vi "Switch Tables.vi"(6 "New Table Name":string, 8 "error in (no error)":errorcluster, 9 "Column Name":string, 10 "Old Table Name":string, 11 "Data.PG":refnum<class "LV-Data.PGSQL.lvclass">) -> (0 "error out":errorcluster, 3 "Data.PG out":refnum<class "LV-Data.PGSQL.lvclass">)   [LabVIEW 2019, in "LV-Data.PGSQL.lvclass"]
uses:
  LV-Data.PGSQL.lvclass
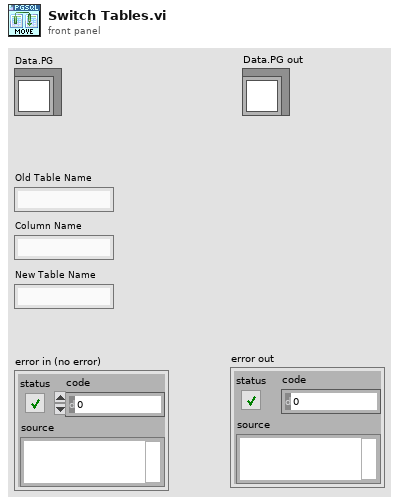
[diagram p1: front panel]
types:
  T1 = enum16{"max points", "1 second", "5 seconds", "10 seconds", "30 seconds", "1 minute", "5 minutes", "10 minutes", "30 minutes", "1 hour", "5 hours", "10 hours", "30 hours"}
  T2 = cluster{"start timestamp":timestamp, "stop timestamp":timestamp}
  T3 = typedef "LV-Data.PGSQL.lvclass/Time.Datatype--enum.ctl" = enum16{"timestamp without time zone", "timestamp with time zone"}
  T4 = typedef "LV-Data.PGSQL.lvclass/Datatypes--enum.ctl" = enum16{"double", "string", "json", "integer", "boolean"}
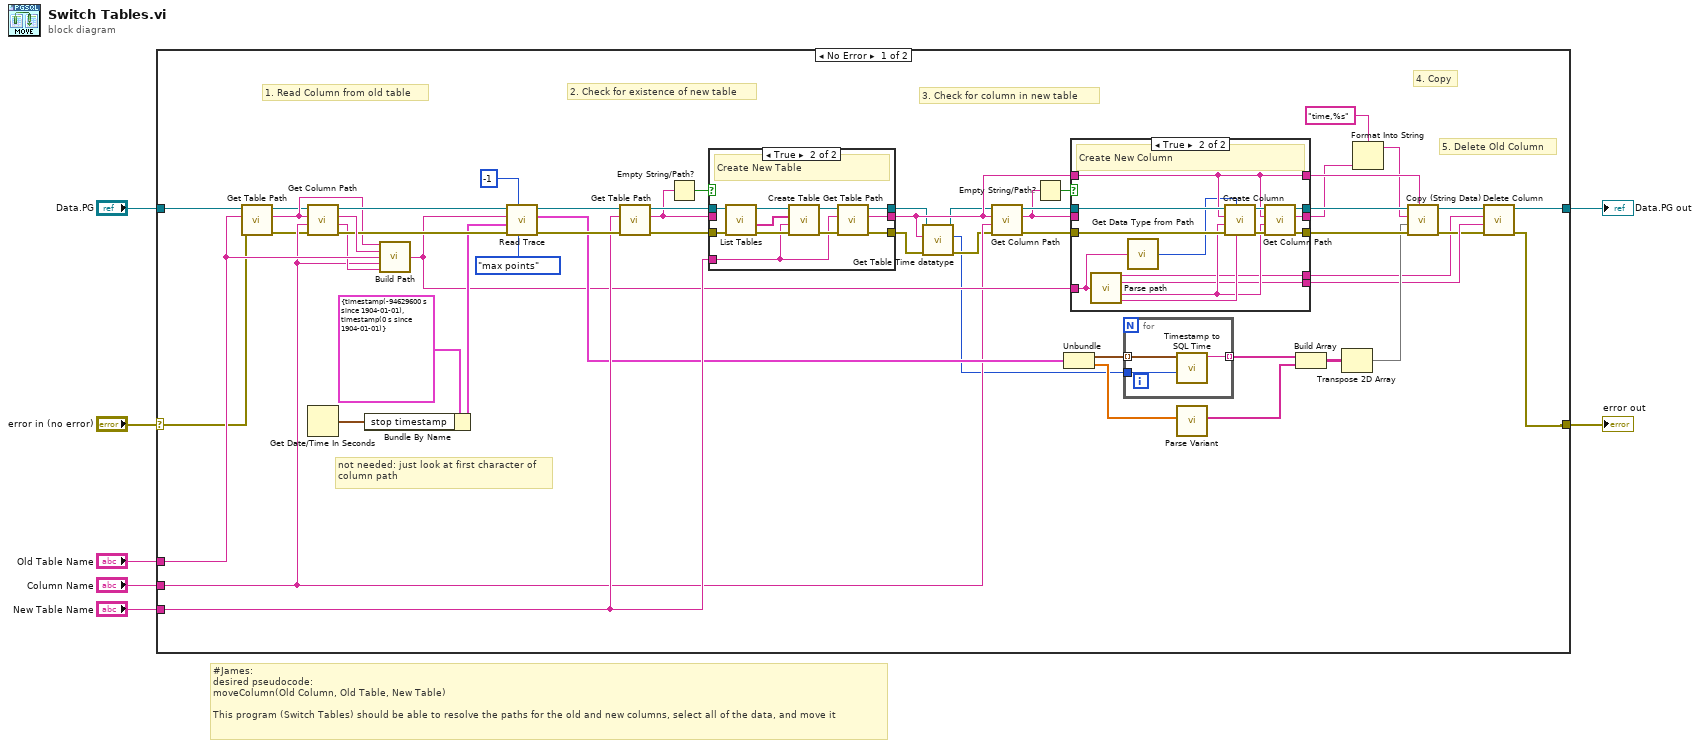
[diagram p0: block diagram]
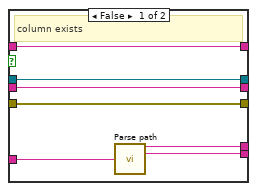
[diagram p3: hidden frame]
diagram:
  # "#James:\ndesired pseudocode:\nmoveColumn(Old Column, Old Table, New Table)\n\nThis program (Switch Tables) should be able to resolve the paths for the old and new columns, select all of the data, and move it"
  n1 = case shown="No Error" "error in (no error)" {
    selector: "error in (no error)" -> [w54 w99]
    tunnel: "New Table Name" -> [w45 _]
    tunnel: "Column Name" -> [w19 _]
    tunnel: "Data.PG" -> [w58 w100]
    tunnel: [w20 w99] -> w1
    tunnel: [w22 w100] -> w5
    tunnel: "Old Table Name" -> [w59 _]
    frame No Error {
      # "4. Copy"
      # "5. Delete Old Column"
      # "3. Check for column in new table"
      # "2. Check for existence of new table"
      # "1. Read Column from old table"
      # "not needed: just look at first character of\ncolumn path"
      n2 = call "Get Table Path.vi"("error in (no error)"=w54, "Table Name"=w59, "Data.PG"=w58) -> ("error out"=w9:errorcluster, "Table Path"=w16:string, "Data.PG out"=w10:refnum<class "LV-Data.PGSQL.lvclass">)  [unwired: 5 in, 1 out]
      n3 = call "Get Column Path.vi"("error in (no error)"=w9, "Column Name"=w19, "Table path"=w16, "Data.PG in"=w10) -> ("error out"=w53:errorcluster, "Column Unit"=w51:string, "Column Path"=w60:string, "Data.PG out"=w57:refnum<class "LV-Data.PGSQL.lvclass">)  [unwired: 4 in]
      n4 = Get Date/Time In Seconds() -> (seconds since 1Jan1904=w55:timestamp)
      n5 = Bundle By Name(cluster=T2 {"start timestamp"=timestamp(-94629600 s since 1904-01-01), "stop timestamp"=timestamp(0 s since 1904-01-01)} ("time interval"), "stop timestamp"=w55) -> (w50:T2)
      n6 = call "Build Path.vi"("Table path"=w16, "Column path"=w60, "Table name"=w59, "Column name"=w19, "Column units"=w51) -> ("PG path"=w29:string)  [unwired: 10 in]
      n7 = call "Read Trace.vi"("time_bucket"=T1."max points", "max points (-1 = all)"=-1 ("max points"), "error in (no error)"=w53, "time interval"=w50, "PG path"=w29, "Data.PGQL in"=w57) -> ("error out"=w49:errorcluster, "Trace"=w38:cluster{timestamp[], dbl[]}, "Data.PGSQL out"=w48:refnum<class "LV-Data.PGSQL.lvclass">)  [unwired: 1 in, 2 out]
      n8 = call "Get Table Path.vi"("error in (no error)"=w49, "Table Name"=w45, "Data.PG"=w48) -> ("error out"=w44:errorcluster, "Table Path"=w43:string, "Data.PG out"=w46:refnum<class "LV-Data.PGSQL.lvclass">)  [unwired: 5 in, 1 out]
      n9 = Empty String/Path?(string/path=w43) -> (empty?=w47:bool)
      n10 = case shown="True" w47 {
        tunnel: w46 -> [w63 w74]
        tunnel: [w63 w65] -> w14
        tunnel: w45 -> [_ w67]
        tunnel: w44 -> [w62 w71]
        tunnel: [w62 w64] -> w12
        tunnel: [w61 w66] -> w15
        tunnel: w43 -> [w61 _]
        frame False {
        }
        frame True {
          # "Create New Table"
          n11 = call "List Tables.vi"("error in (no error)"=w71, "Data.PG"=w74) -> ("error out"=w70:errorcluster, "Table Paths"=w72:string[], "Data.PG"=w73:refnum<class "LV-Data.PGSQL.lvclass">)  [unwired: 6 in, 1 out]
          n12 = call "Create Table.vi"("error in (no error)"=w70, "New Table Name"=w67, "Table Paths"=w72, "Data.PGSQL"=w73) -> ("error out"=w68:errorcluster, "Data.PGSQL out"=w69:refnum<class "LV-Data.PGSQL.lvclass">)  [unwired: 6 in]
          n13 = call "Get Table Path.vi"("error in (no error)"=w68, "Table Name"=w67, "Data.PG"=w69) -> ("error out"=w64:errorcluster, "Table Path"=w66:string, "Data.PG out"=w65:refnum<class "LV-Data.PGSQL.lvclass">)  [unwired: 5 in, 1 out]
        }
      }
      n14 = call "Get Table Time datatype.vi"("error in (no error)"=w12, "Table path"=w15, "LV-Data.PGSQL in"=w14) -> ("error out"=w11:errorcluster, "Time Datatype"=w8:T3, "LV-Data.PGSQL out"=w13:refnum<class "LV-Data.PGSQL.lvclass">)  [unwired: 6 in]
      n15 = call "Get Column Path.vi"("error in (no error)"=w11, "Column Name"=w19, "Table path"=w15, "Data.PG in"=w13) -> ("error out"=w40:errorcluster, "Column Path"=w39:string, "Data.PG out"=w41:refnum<class "LV-Data.PGSQL.lvclass">)  [unwired: 4 in, 1 out]
      n16 = Empty String/Path?(string/path=w39) -> (empty?=w42:bool)
      n17 = Unbundle(w38) -> (w35:timestamp[], w34:dbl[])
      n18 = case shown="True" w42 {
        tunnel: w41 -> [w84 w97]
        tunnel: [w84 w93] -> w36
        tunnel: w40 -> [w83 w98]
        tunnel: [w83 w91] -> w30
        tunnel: w15 -> [w82 w86]
        tunnel: w29 -> [w80 w89]
        tunnel: [w82 w86] -> w37
        tunnel: [w81 w95] -> w27
        tunnel: w39 -> [w81 _]
        tunnel: [w79 w88] -> w23
        tunnel: [w78 w87] -> w17
        frame False {
          # "column exists"
          n19 = call "Parse path.vi"("PG Path"=w80) -> ("Table path"=w78:string, "Column path"=w79:string)  [unwired: 10 in, 3 out]
        }
        frame True {
          # "Create New Column"
          n20 = call "Parse path.vi"("PG Path"=w89) -> ("Table path"=w87:string, "Column path"=w88:string, "Column name"=w90:string, "Column units"=w96:string)  [unwired: 10 in, 1 out]
          n21 = call "Get Data Type from Path.vi"("PG Path"=w89) -> ("data type"=w85:T4)
          n22 = call "Create Column.vi"("new column units"=w96, "Data type"=w85, "error in (no error)"=w98, "new column name"=w90, "selected table path"=w86, "Data.PGSQL in"=w97) -> ("error out"=w92:errorcluster, "Data.PGSQL out"=w94:refnum<class "LV-Data.PGSQL.lvclass">)  [unwired: 4 in]
          n23 = call "Get Column Path.vi"("error in (no error)"=w92, "Column Name"=w90, "Table path"=w86, "Data.PG in"=w94) -> ("error out"=w91:errorcluster, "Column Path"=w95:string, "Data.PG out"=w93:refnum<class "LV-Data.PGSQL.lvclass">)  [unwired: 4 in, 1 out]
        }
      }
      n24 = for {
        tunnel: w35 -> [w77] mode=indexing
        tunnel: [w76] -> w33 mode=indexing
        tunnel: w8 -> [w75]
        n25 = call "Timestamp to SQL Time.vi"("Time Datatype"=w75, "Timestamp"=w77) -> ("date/time string"=w76:string)  [unwired: 9 in]
      }
      n26 = call "Parse Variant.vi"("Data"=w34) -> ("Data"=w32:string[])  [unwired: 6 in, 4 out]
      n27 = Build Array(w33, w32) -> (w31:string[][])
      n28 = Transpose 2D Array(2D array=w31) -> (transposed array=w28:string[][])
      n29 = Format Into String(format string="time,%s", w27) -> (resulting string=w26:string)  [unwired: 2 in, 1 out]
      n30 = call "Copy (String Data).vi"("table \"path\""=w37, "error in (no error)"=w30, "data"=w28, "column \"path\"(s) (empty=ALL)"=w26, "Data.PGSQL"=w36) -> ("error out"=w21:errorcluster, "Data.PGSQL out"=w24:refnum<class "LV-Data.PGSQL.lvclass">)  [unwired: 5 in]
      n31 = call "Delete Column.vi"("error in"=w21, "Column path"=w23, "Table Path"=w17, "LV-Data.PG"=w24) -> ("error out"=w20:errorcluster, "LV-Data.PG out"=w22:refnum<class "LV-Data.PGSQL.lvclass">)  [unwired: 6 in]
    }
    frame Error {
    }
  }
  "Data.PG out" <- w5
  "error out" <- w1
